vi "Read Moving Flags.vi"(8 "error in (no error)":errorcluster, 11 "XY Stage Controller in":refnum<class "XY Stage Controller.lvclass">) -> (0 "error out":errorcluster, 1 "Y-Axis Moving":bool, 2 "X-Axis Moving":bool, 3 "XY Stage Controller out":refnum<class "XY Stage Controller.lvclass">)   [LabVIEW 2022 SP3, in "XY Stage Controller.lvclass"]
uses:
  XY Stage Controller.lvclass
  XY Stage Data Class/XY Stage Data Class.lvclass
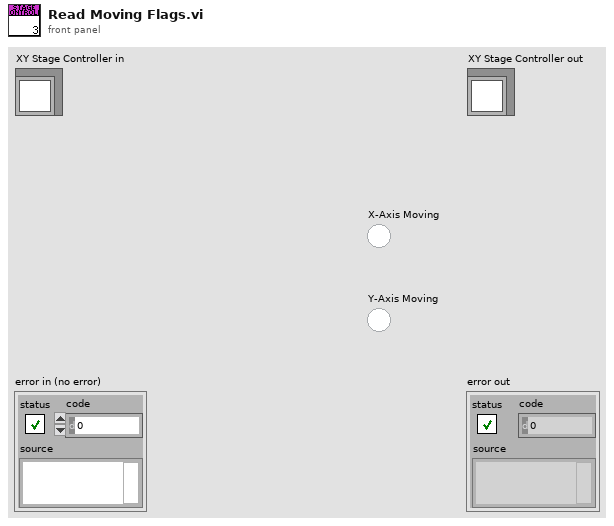
[diagram p1: front panel]
types:
  T1 = typedef "XY Stage Data Class.lvclass/Moving.ctl" = cluster{"X Moving":bool, "Y Moving":bool}
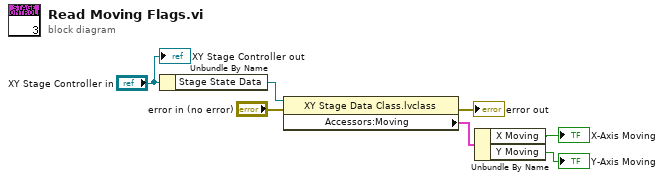
[diagram p0: block diagram]
diagram:
  n1 = Unbundle By Name("XY Stage Controller in") -> ("Stage State Data"=w6:refnum<data-value>)
  n2 = property class="XY Stage Data Class.lvclass"(reference=w6, error in="error in (no error)") -> (error out=→"error out":errorcluster, "Accessors:Moving"=w3:T1)  [unwired: 1 out]
  n3 = Unbundle By Name(w3) -> ("X Moving"=→"X-Axis Moving":bool, "Y Moving"=→"Y-Axis Moving":bool)
  "XY Stage Controller out" <- "XY Stage Controller in"
